vi "Flip Transform-Matrix Handedness.vi"(1 "Transform Matrix in":T1) -> (0 "Transform Matrix out":T1)   [LabVIEW 2020, in "g_ar_toolkit.ar.lvlib"]
uses:
  g_ar_toolkit.ar.lvlib
  <vilib>/Analysis/NI_AALBase.lvlib
  <vilib>/Analysis/baseanly.llb/Real A x B.vi
  <vilib>/Analysis/Matrix/Datatypes/RealMatrix.ctl
  <vilib>/Analysis/Matrix/NI_Matrix.lvlib
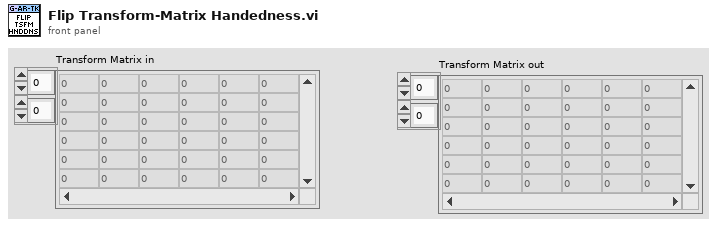
[diagram p1: front panel]
types:
  T1 = typedef "NI_Matrix.lvlib/RealMatrix.ctl" = dbl[][]
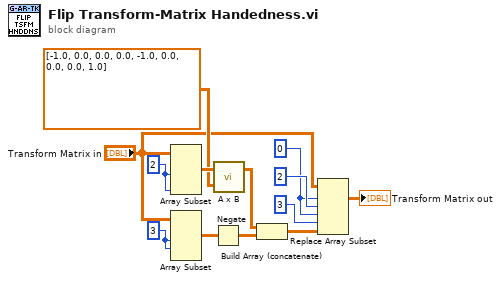
[diagram p0: block diagram]
diagram:
  w2 = 0 ("row 1")
  w7 = 3 ("disabled index (col)")
  w9 = 2 ("row N")
  n1 = Array Subset(array="Transform Matrix in", length (row)=w9, length (col)=w9) -> (w12:T1)  [unwired: 2 in]
  n2 = Array Subset(array="Transform Matrix in", length (row)=w7, index (col)=w7) -> (w13:T1)  [unwired: 2 in]
  n3 = Negate(x=w13) -> (-x=w8:T1)
  n4 = call-poly <vilib>:"A x B.vi"("B"=T1 [[-1.0, 0.0, 0.0], [0.0, -1.0, 0.0], [0.0, 0.0, 1.0]], "A"=w12) -> ("A x B"=w11:T1)  [unwired: 1 out]
  n5 = Build Array (concatenate)(w11, w8) -> (w5:T1)
  n6 = Replace Array Subset(array="Transform Matrix in", new element=w5, index (dim 0)=w2, index (dim 1)=2 ("row N"), index (dim 2)=w2, index (dim 3)=3 ("column N")) -> (→"Transform Matrix out":T1)
